vi "CRYIs Empty Asio Device.vi"(11 "Device Info":T1(array[cluster])) -> (3 "IsEmptyASIO":bool)   [LabVIEW 2013]
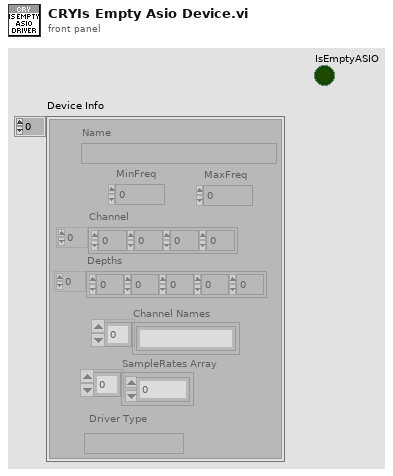
[diagram p1: front panel]
types:
  T1 = cluster{"Name":string, "MinFreq":dbl, "MaxFreq":dbl, "Channel":i32[], "Depths":i32[], "Channel Names":string[], "SampleRates Array":dbl[], "Driver Type":string}[]
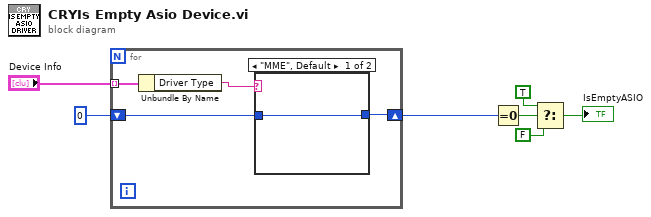
[diagram p0: block diagram]
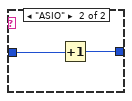
[diagram p2: hidden frame]
diagram:
  n1 = for {
    tunnel: "Device Info" -> [w11] mode=indexing
    shift-right: [w8] -> w5
    shift-left: 0 -> [w9]
    n2 = Unbundle By Name(w11) -> ("Driver Type"=w10:string)
    n3 = case shown="\"MME\", Default" w10 {
      tunnel: w9 -> [w12 w14]
      tunnel: [w12 w13] -> w8
      frame "MME", Default {
      }
      frame "ASIO" {
        n4 = Increment(x=w14) -> (x+1=w13:i32)
      }
    }
  }
  n5 = Equal To 0?(x=w5) -> (x = 0?=w4:bool)
  n6 = Select(t=TRUE ("x = 0?"), s=w4, f=FALSE ("x = 0?")) -> (s? t:f=→"IsEmptyASIO":bool)
